vi "Main.vi"() -> ()   [LabVIEW 2019]
uses:
  Typedefs/#enum_MasterState.ctl
  <vilib>/ActorFramework/Message Enqueuer/Message Enqueuer.lvclass
  Typedefs/#cluster_GUIRefs.ctl
  <vilib>/ActorFramework/Message Enqueuer/Message Enqueuer.lvclass/Message Enqueuer.ctl
  ResultsViewer/ResultsViewer/ResultsViewer.lvclass
  C:/Program Files (x86)/National Instruments/LabVIEW 2019/vi.lib/ActorFramework/Actor/Actor.lvclass
  SubVIs/Application Configuration VIs/#cluster_AppConfiguration.ctl
  <vilib>/ActorFramework/Message Enqueuer/Enqueue.vi
  <vilib>/ActorFramework/Stop Msg/Stop Msg.lvclass
  C:/Program Files (x86)/National Instruments/LabVIEW 2019/vi.lib/ActorFramework/Message/Message.lvclass
  <vilib>/ActorFramework/Message Priority Queue/Priority Enqueue.vi
  SubVIs/LowLevelError.vi
  <vilib>/ActorFramework/Actor/Actor.lvclass
panel:
  in  "Results Viewer":bool
  in  "POX Data History":string[](array[string])
  in  "Save?":bool caption="Save Results?"
  in  "Measure":bool
  in  "Measurement Directory":path
  in  "Stop":bool
  out "O2 Saturation":dbl(graph)
  out "Heart beat":dbl(graph)
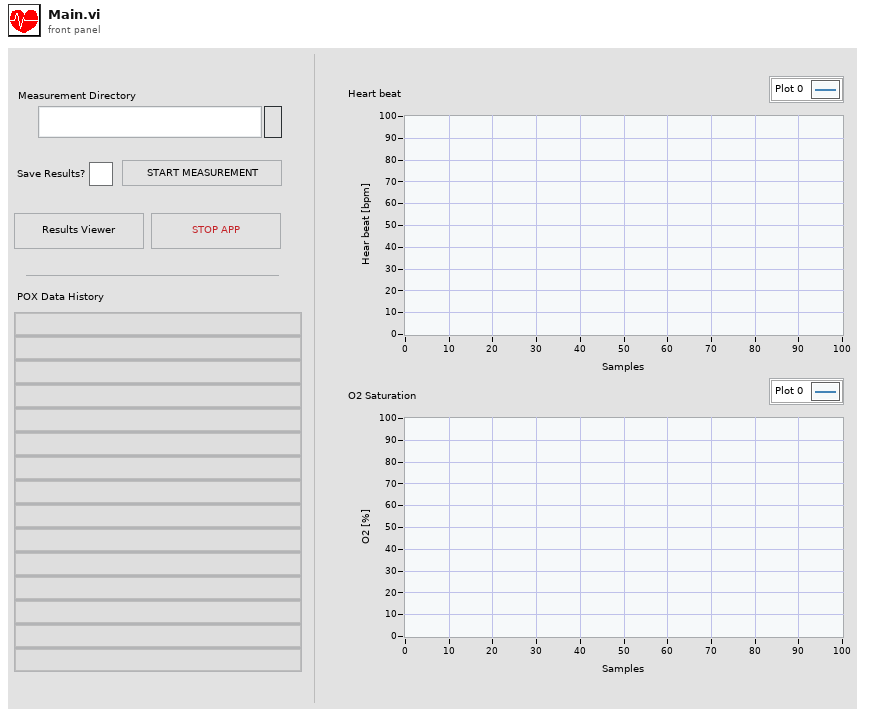
[diagram p1: front panel]
types:
  T1 = typedef "#enum_MasterState.ctl" = enum16{"Idle", "Init", "Close", "Error"}
  T2 = typedef "#cluster_ApplicationData.ctl" = cluster{"Acq Queue":refnum<queue>, "Saving Queue":refnum<queue>, "Launched Viewers":refnum<class "Message Enqueuer.lvclass">[]}
  T3 = typedef "#cluster_GUIRefs.ctl" = cluster{"Measure":refnum<vi>, "Save?":refnum<vi>, "Stop":refnum<vi>, "Measurement Dir":refnum<vi>, "Heart beat":refnum<vi>, "O2":refnum<vi>, "POX Data History":refnum<vi>}
  T4 = typedef "#cluster_AppConfiguration.ctl" = cluster{"Measurements Directory":path}
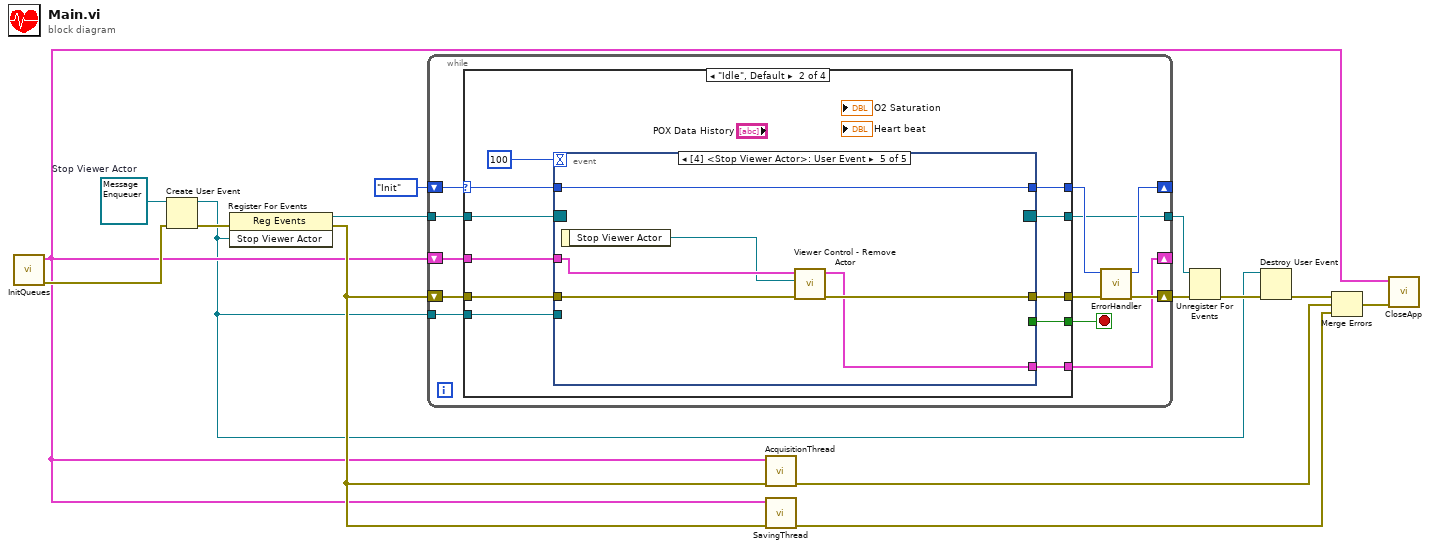
[diagram p0: block diagram]
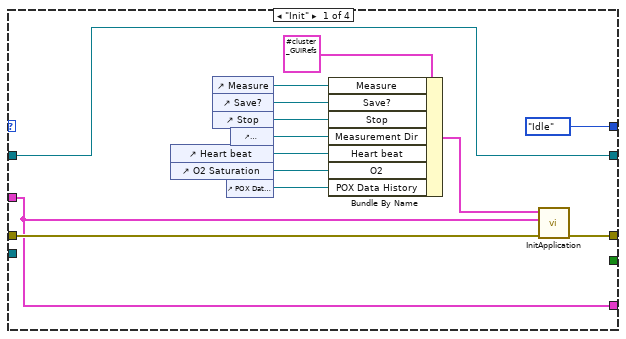
[diagram p2: hidden frame]
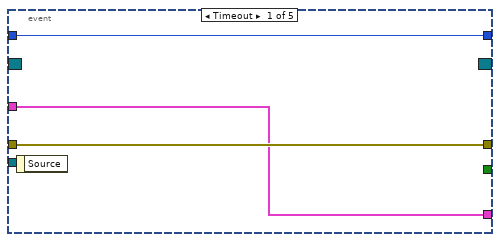
[diagram p3: hidden frame]
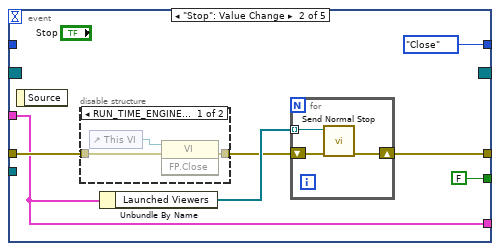
[diagram p4: hidden frame]
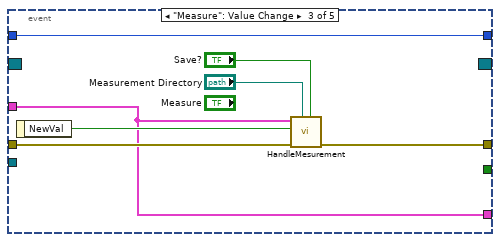
[diagram p6: hidden frame]
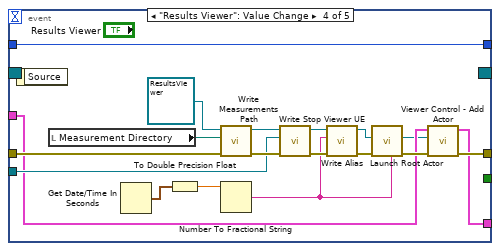
[diagram p7: hidden frame]
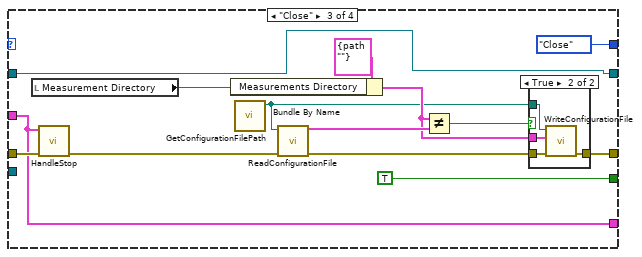
[diagram p8: hidden frame]
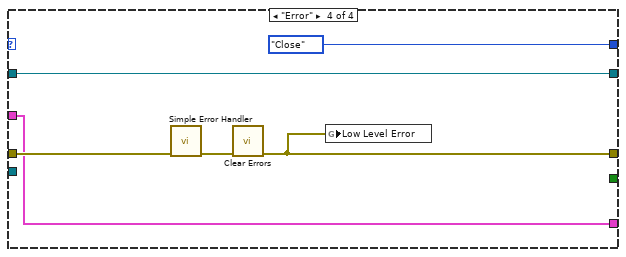
[diagram p10: hidden frame]
diagram:
  w8 = refnum<class "Message Enqueuer.lvclass"> refnum  # Stop Viewer Actor
  n1 = call "InitQueues.vi"() -> ("error out"=w7:errorcluster, "Application Data"=w6:T2)  [unwired: 10 in]
  n2 = Create User Event(user event datatype=w8, error in=w7) -> (user event=w1:refnum<user-event>, error out=w11:errorcluster)
  n3 = register-events(error in=w11, w1) -> (reference out=w10:refnum<event-registration>, error out=w9:errorcluster)  [unwired: 1 in]
  n4 = while {
    shift-right: [w22] -> w15
    shift-left: w9 -> [w27]
    shift-right: [w20] -> _
    shift-left: #enum_MasterState."Init" ("Master State") -> [w24]
    tunnel: w10 -> [w19]
    tunnel: w1 -> [w18]
    shift-right: [w17] -> _
    shift-left: w6 -> [w26]
    tunnel: [w16] -> w3
    stop <- w25 stop-if-true
    n5 = case shown="\"Idle\", Default" w24 {
      selector: w24 -> [_ w49 _ _]
      tunnel: w27 -> [w34 w52 w115 w125]
      tunnel: w26 -> [w29 w44 w103 w122]
      tunnel: [w32 w51 w109 w123] -> w23
      tunnel: [_ w50 TRUE _] -> w25
      tunnel: [#enum_MasterState."Idle" ("Master State") w48 #enum_MasterState."Close" ("Master State") #enum_MasterState."Close" ("Master State")] -> w21
      tunnel: w19 -> [w28 w46 w102 w121]
      tunnel: w18 -> [_ w45 _ _]
      tunnel: [w29 w43 w103 w122] -> w17
      tunnel: [w28 w42 w102 w121] -> w16
      frame "Init" {
        n6 = control-ref of="Heart beat"() -> (w40:refnum<vi>)
        n7 = control-ref of="O2 Saturation"() -> (w41:refnum<vi>)
        n8 = control-ref of="Measure"() -> (w36:refnum<vi>)
        n9 = control-ref of="Save?"() -> (w37:refnum<vi>)
        n10 = control-ref of="Stop"() -> (w38:refnum<vi>)
        n11 = control-ref of="POX Data History"() -> (w30:refnum<vi>)
        n12 = control-ref of="Measurement Directory"() -> (w39:refnum<vi>)
        n13 = Bundle By Name(cluster=T3 {"Measure"=refnum, "Save?"=refnum, "Stop"=refnum, "Measurement Dir"=refnum, "Heart beat"=refnum, "O2"=refnum, "POX Data History"=refnum} ("GUI Refs"), "Measure"=w36, "Save?"=w37, "Stop"=w38, "Measurement Dir"=w39, "Heart beat"=w40, "O2"=w41, "POX Data History"=w30) -> (w33:T3)
        n14 = call "InitApplication.vi"("error in (no error)"=w34, "Application Data in"=w29, "GUI Refs"=w33) -> ("error out"=w32:errorcluster)  [unwired: 8 in]
      }
      frame "Idle", Default {
        n15 = event shown="[4] <Stop Viewer Actor>: User Event" {
          selector: w46 -> [_ _ _ _ _]
          dyn-events: [_ _ _ _ _] -> w42
          timeout: 100 -> [_ _ _ _ _]
          tunnel: w52 -> [w55 w62 w76 w95 w101]
          tunnel: w44 -> [w53 w59 w70 w86 w99]
          tunnel: [w55 w56 w74 w87 w100] -> w51
          tunnel: [_ FALSE _ _ _] -> w50
          tunnel: w49 -> [w54 _ w71 w83 w96]
          tunnel: [w54 #enum_MasterState."Close" ("Master State") w71 w83 w96] -> w48
          tunnel: w45 -> [_ _ _ w88 _]
          tunnel: [w53 w59 w70 w84 w97] -> w43
          event Timeout {
            n16 = event-data() -> ()  [unwired: 1 in, 1 out]
          }
          event "Stop": Value Change {
            n17 = event-data() -> ()  [unwired: 1 in, 1 out]
            n18 = disable-structure shown="RUN_TIME_ENGINE==True" {
              disable-tunnel: w62 -> [w68 w69]
              disable-tunnel: [w67 w69] -> w57
              frame condition #0 {
                n19 = control-ref of="This VI"() -> (w66:refnum<vi>)
                n20 = invoke class="VI" method="FP.Close"(reference=w66, error in=w68) -> (error out=w67:errorcluster)  [unwired: 1 in, 2 out]
              }
              frame condition #1 (active) {
              }
            }
            n21 = Unbundle By Name(w59) -> ("Launched Viewers"=w58:refnum<class "Message Enqueuer.lvclass">[])
            n22 = for {
              tunnel: w58 -> [w65] mode=indexing
              shift-right: [w63] -> w56
              shift-left: w57 -> [w64]
              n23 = call <vilib>:"Send Normal Stop.vi"("error in (no error)"=w64, "Message Enqueuer"=w65) -> ("error out"=w63:errorcluster)  [unwired: 9 in]
            }
          }
          event "Measure": Value Change {
            n24 = event-data() -> ("NewVal"=w75:bool)  [unwired: 1 in]
            n25 = call "HandleMesurement.vi"("Save?"="Save?", "Measurement Directory"="Measurement Directory", "error in (no error)"=w76, "Measure?"=w75, "Application Data"=w70) -> ("error out"=w74:errorcluster)  [unwired: 6 in]
          }
          event "Results Viewer": Value Change {
            n26 = event-data() -> ()  [unwired: 1 in, 1 out]
            n27 = local read "Measurement Directory"() -> (w91:path)
            n28 = Get Date/Time In Seconds() -> (seconds since 1Jan1904=w82:timestamp)
            n29 = To Double Precision Float(number=w82) -> (double precision float=w77:dbl)
            n30 = call-dynamic "Write Measurements Path.vi"("error in (no error)"=w95, "Measurements Path"=w91, "ResultsViewer in"=refnum<class "ResultsViewer.lvclass"> refnum ("ResultsViewer.lvlib:ResultsViewer.lvclass")) -> ("error out"=w93:errorcluster, "ResultsViewer out"=w89:refnum<class "ResultsViewer.lvclass">)  [unwired: 7 in]
            n31 = Number To Fractional String(number=w77) -> (F-format string=w78:string)  [unwired: 3 in]
            n32 = call-dynamic "Write Stop Viewer UE.vi"("error in (no error)"=w93, "Stop Viewer UE"=w88, "ResultsViewer in"=w89) -> ("error out"=w90:errorcluster, "ResultsViewer out"=w80:refnum<class "ResultsViewer.lvclass">)  [unwired: 7 in]
            n33 = call-dynamic "Write Alias.vi"("error in (no error)"=w90, "Alias"=w78, "ResultsViewer in"=w80) -> ("error out"=w81:errorcluster, "ResultsViewer out"=w79:refnum<class "ResultsViewer.lvclass">)  [unwired: 7 in]
            n34 = call <vilib>:"Launch Root Actor.vi"("Debug Alias"=w78, "error in (no error)"=w81, "Actor"=w79) -> ("error out"=w94:errorcluster, "Actor's Enqueuer"=w85:refnum<class "Message Enqueuer.lvclass">)  [unwired: 7 in]
            n35 = call "Viewer Control - Add Actor.vi"("error in"=w94, "Stop Viewer Actor"=w85, "App Data in"=w86) -> ("error out"=w87:errorcluster, "App Data out"=w84:T2)  [unwired: 7 in]
          }
          event User Event {
            n36 = event-data() -> ("Stop Viewer Actor"=w98:refnum<class "Message Enqueuer.lvclass">)  [unwired: 1 in]
            n37 = call "Viewer Control - Remove Actor.vi"("error in"=w101, "Stop Viewer Actor"=w98, "App Data in"=w99) -> ("error out"=w100:errorcluster, "App Data out"=w97:T2)  [unwired: 7 in]
          }
        }
      }
      frame "Close" {
        n38 = local read "Measurement Directory"() -> (w107:path)
        n39 = call "HandleStop.vi"("error in (no error)"=w115, "Application Data"=w103) -> ("error out"=w112:errorcluster)  [unwired: 9 in]
        n40 = Bundle By Name(cluster=T4 {"Measurements Directory"=path ""} ("App Configuration"), "Measurements Directory"=w107) -> (w105:T4)
        n41 = call "GetConfigurationFilePath.vi"() -> ("Configuration File Path"=w104:path)  [unwired: 11 in]
        n42 = call "ReadConfigurationFile.vi"("Error in"=w112, "Configuration File Path"=w104) -> ("Error out"=w111:errorcluster, "App Configuration"=w106:T4)  [unwired: 8 in]
        n43 = Not Equal?(x=w105, y=w106) -> (x != y?=w110:bool)
        n44 = case shown="True" w110 {
          tunnel: w111 -> [w116 w120]
          tunnel: [w116 w119] -> w109
          tunnel: w105 -> [_ w118]
          tunnel: w104 -> [_ w117]
          frame False {
          }
          frame True {
            n45 = call "WriteConfigurationFile.vi"("Error in"=w120, "App Configuration"=w118, "Configuration File Path"=w117) -> ("Error out"=w119:errorcluster)  [unwired: 8 in]
          }
        }
      }
      frame "Error" {
        n46 = call <vilib>:"Simple Error Handler.vi"("error in (no error)"=w125) -> ("error out"=w124:errorcluster)  [unwired: 4 in, 4 out]
        n47 = call <vilib>:"Clear Errors.vi"("error in (no error)"=w124) -> ("error out"=w123:errorcluster)  [unwired: 5 in, 1 out]
        n48 = global write "LowLevelError.vi" "Low Level Error"(w123) -> ()
      }
    }
    n49 = call "ErrorHandler.vi"("error in (no error)"=w23, "Master State in"=w21) -> ("error out"=w22:errorcluster, "Master State out"=w20:T1)  [unwired: 8 in]
  }
  n50 = call "AcquisitionThread.vi"("error in (no error)"=w9, "Application Data"=w6) -> ("error out"=w14:errorcluster)  [unwired: 9 in]
  n51 = call "SavingThread.vi"("error in (no error)"=w9, "Application Data"=w6) -> ("error out"=w12:errorcluster)  [unwired: 9 in]
  n52 = Unregister For Events(event registration refnum=w3, error in=w15) -> (error out=w4:errorcluster)
  n53 = Destroy User Event(user event=w1, error in=w4) -> (error out=w2:errorcluster)
  n54 = Merge Errors(w2, w14, w12) -> (w5:errorcluster)
  n55 = call "CloseApp.vi"("error in (no error)"=w5, "Application Data"=w6) -> ()  [unwired: 9 in, 1 out]
